vi "数字输出_有限.vi"() -> ()   [LabVIEW 2013]
doc: "This example demonstrates how to read values from a digital input port."
uses:
  <userlib>/ArtDAQ/_SubVI/ArtDAQ_CreateDOChan.vi
  <userlib>/ArtDAQ/_SubVI/ArtDAQ_CfgSampClkTiming.vi
  <userlib>/ArtDAQ/_SubVI/ArtDAQ_Write Digital Bool NChan NSamp.vi
  <userlib>/ArtDAQ/_SubVI/ArtDAQ_CfgDigEdgeStartTrig.vi
panel:
  in  "?":bool[][](array[boolean])=[[TRUE, FALSE, TRUE, FALSE], [FALSE, FALSE, FALSE, FALSE], [FALSE, TRUE, FALSE, TRUE]]
  out "错误输出":errorcluster
  in  "触发模式":enum32{"无触发", "数字边沿"}(tab)
  in  "有效边沿":i32(ring)=10280 items=["上升"=10280, "下降"=10171]
  in  "触发源":string
  in  "每通道采样数":i32=40
  in  "采样速率":dbl=100.0
  in  "时钟源":string="/Dev1/PFI0"
  in  "端口":string="Dev1/port0/line0:2"
  # "通道属性"
  # "定时"
  # "触发"
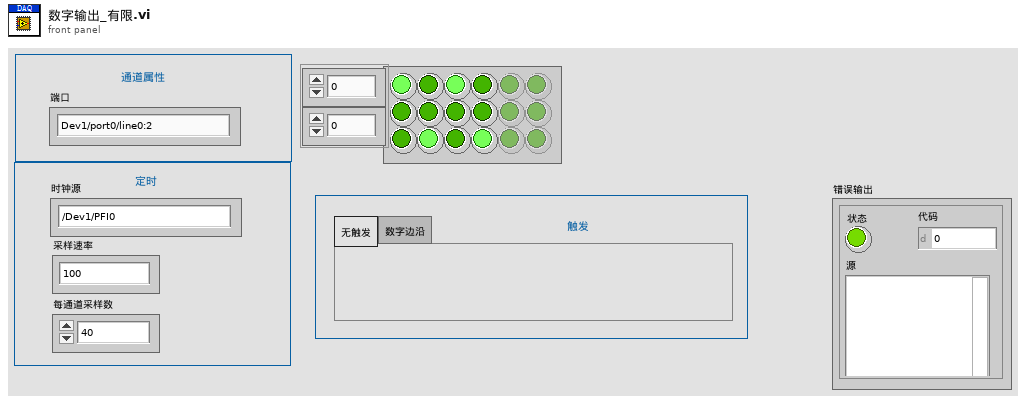
[diagram p1: front panel]
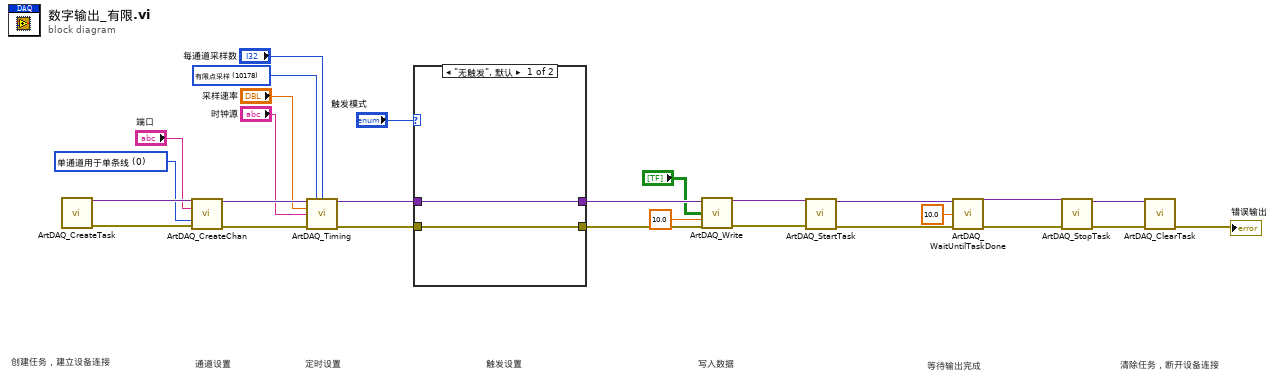
[diagram p0: block diagram]
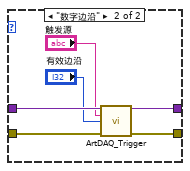
[diagram p2: hidden frame]
diagram:
  w17 = 10178 items=["有限点采样"=10178, "连续采样"=10123] ("SampleMode")
  w22 = 0 items=["单通道用于单条线", "单通道用于所有线"] ("Line Grouping")
  # "清除任务，断开设备连接"
  # "等待输出完成"
  # "写入数据"
  # "触发设置"
  # "定时设置"
  # "通道设置"
  # "创建任务，建立设备连接"
  n1 = call <userlib>:"ArtDAQ_CreateTask.vi"() -> ("任务句柄"=w27:variant, "错误输出"=w26:errorcluster)  [unwired: 14 in]
  n2 = call-poly <userlib>:"ArtDAQ_CreateChan.vi"("任务句柄"=w27, "线"="端口", "线分组"=w22, "错误输入"=w26) -> ("任务句柄"=w20:variant, "错误输出"=w21:errorcluster)  [unwired: 10 in]
  n3 = call-poly <userlib>:"ArtDAQ_Timing.vi"("任务句柄"=w20, "采样模式"=w17, "每通道采样数"="每通道采样数", "采样率"="采样速率", "源"="时钟源", "错误输入"=w21) -> ("任务句柄"=w15:variant, "错误输出"=w14:errorcluster)  [unwired: 8 in]
  n4 = case shown="\"无触发\", 默认" "触发模式" {
    tunnel: w15 -> [w29 w35]
    tunnel: w14 -> [w28 w34]
    tunnel: [w29 w33] -> w9
    tunnel: [w28 w32] -> w12
    frame "无触发", Default {
    }
    frame "数字边沿" {
      n5 = call-poly <userlib>:"ArtDAQ_Trigger.vi"("任务句柄"=w35, "触发源"="触发源", "边沿"="有效边沿", "错误输入"=w34) -> ("任务句柄"=w33:variant, "错误输出"=w32:errorcluster)  [unwired: 10 in]
    }
  }
  n6 = call-poly <userlib>:"ArtDAQ_Write.vi"("任务句柄"=w9, "数据"="?", "超时s"=10.0 ("Timeout"), "错误输入"=w12) -> ("任务句柄"=w10:variant, "错误输出"=w11:errorcluster)  [unwired: 9 in, 1 out]
  n7 = call <userlib>:"ArtDAQ_StartTask.vi"("任务句柄"=w10, "错误输入"=w11) -> ("任务句柄"=w2:variant, "错误输出"=w1:errorcluster)  [unwired: 12 in]
  n8 = call <userlib>:"ArtDAQ_WaitUntilTaskDone.vi"("任务输入"=w2, "超时s"=10.0 ("TimeToWait"), "错误输入"=w1) -> ("任务输出"=w4:variant, "错误输出"=w3:errorcluster)  [unwired: 11 in]
  n9 = call <userlib>:"ArtDAQ_StopTask.vi"("任务句柄"=w4, "错误输入"=w3) -> ("任务句柄"=w24:variant, "错误输出"=w25:errorcluster)  [unwired: 12 in]
  n10 = call <userlib>:"ArtDAQ_ClearTask.vi"("任务句柄"=w24, "错误输入"=w25) -> ("错误输出"=→"错误输出":errorcluster)  [unwired: 13 in]
